vi "Realback.vi"() -> ()   [LabVIEW 2013]
uses:
  <vilib>/Utility/file.llb/Read From Spreadsheet File (DBL).vi
panel:
  in  "# skip":i32
  in  "# of sweeps":i32=1000
  out "Spectrum #":i32=999
  out "Chars":i32=1282716
  out "Fcen":dbl=213.0 format="%#_13g"
  out "# Data points":i32=101
  in  "Offset V":dbl format="%#_3g"
  out "NMR Graph + Fit":cluster{dbl, dbl}[](graph)=[{212.6, -0.16073883883883802}, {212.608, -0.16040180180180247}, {212.61599999999999, -0.1600734734734744}, {212.624, -0.1597480480480463}, {212.632, -0.1594280280280284}, {212.64, -0.15912582582582555}, {212.648, -0.15882072072072065}, {212.656, -0.158519319319321}, {212.664, -0.15823073073073043}, {212.672, -0.1579462462462453}, {212.68, -0.15766146146146215}, {212.688, -0.1573662662662664}, {212.696, -0.1570670670670683}, {212.704, -0.15675385385385404}, {212.712, -0.1564493493493483}, {212.72, -0.1561526526526524}, {212.728, -0.15587627627627706}, {212.736, -0.1556206206206206}, {212.744, -0.1553856856856856}, {212.752, -0.15515845845845858}, {212.76, -0.1549458458458459}, {212.768, -0.15473903903903835}, {212.776, -0.15453673673673607}, {212.784, -0.15433903903903998}, {212.792, -0.15414684684684804}, {212.79999999999998, -0.15395325325325318}, {212.808, -0.15376576576576428}, {212.816, -0.15358708708708604}, {212.82399999999998, -0.1534129129129131}, {212.832, -0.1532410410410411}, {212.84, -0.1530826826826821}, {212.84799999999998, -0.1529271271271264}, {212.856, -0.15278578578578608}, {212.864, -0.1526609609609621}, {212.87199999999999, -0.15253163163163322}, {212.88, -0.15241391391391546}, {212.888, -0.15231491491491583}, {212.896, -0.15221491491491465}, {212.904, -0.15212162162162043}, {212.912, -0.1520264264264249}, {212.92, -0.15195275275275122}, {212.928, -0.15188108108107995}, {212.936, -0.15181641641641605}, {212.944, -0.15176516516516494}, {212.952, -0.15173403403403407}, {212.96, -0.15173313313313336}, {212.968, -0.15177017017016978}, {212.976, -0.1518006006006003}, {212.984, -0.15173983983984016}, {212.992, -0.15169779779779818}, {213.0, -0.1516902902902905}, {213.008, -0.15169489489489518}, {213.016, -0.15168108108108158}, {213.024, -0.15169089089089133}, {213.032, -0.15172112112112154}, {213.04, -0.15176556556556584}, {213.048, -0.15179779779779762}, {213.056, -0.15185625625625562}, {213.064, -0.15193223223223107}, {213.072, -0.15198738738738587}, {213.08, -0.15204724724724555}, {213.088, -0.15212502502502398}, {213.096, -0.1522167167167166}, {213.104, -0.15231871871871952}, {213.112, -0.15243293293293445}, {213.12, -0.15255175175175337}, {213.12800000000001, -0.1526766766766775}, {213.136, -0.15282012012011958}, {213.144, -0.1529715715715709}, {213.15200000000002, -0.1531350350350349}, {213.16, -0.1533186186186189}, {213.168, -0.15351111111111057}, {213.17600000000002, -0.15370180180180038}, {213.184, -0.15391111111111092}, {213.192, -0.15412052052052155}, {213.2, -0.15434864864864928}, {213.208, -0.1545821821821811}, {213.216, -0.15481641641641614}, {213.224, -0.15505325325325345}, {213.232, -0.15529939939939943}, {213.24, -0.1555706706706705}, {213.248, -0.1558586586586596}, {213.256, -0.15617497497497437}, {213.264, -0.15652822822822776}, {213.272, -0.1569007007007014}, {213.28, -0.15727547547547563}, {213.288, -0.15764314314314382}, {213.296, -0.15800110110109958}, {213.304, -0.15834644644644752}, {213.312, -0.1587058058058067}, {213.32, -0.15907317317317304}, {213.328, -0.15945115115115094}, {213.336, -0.15984504504504424}, {213.344, -0.16024984984985124}, {213.352, -0.1606673673673666}, {213.36, -0.16110060060060055}, {213.368, -0.1615386386386386}, {213.376, -0.16198208208208292}, {213.38400000000001, -0.16242522522522437}, {213.392, -0.16287507507507482}, {213.4, -0.16338568568568626}]
  out "File size (bytes)":i32=1284000
  out "File name":string="C:\\Users\\plm\\Desktop\\rssmt\\NMR3494011168.xls"
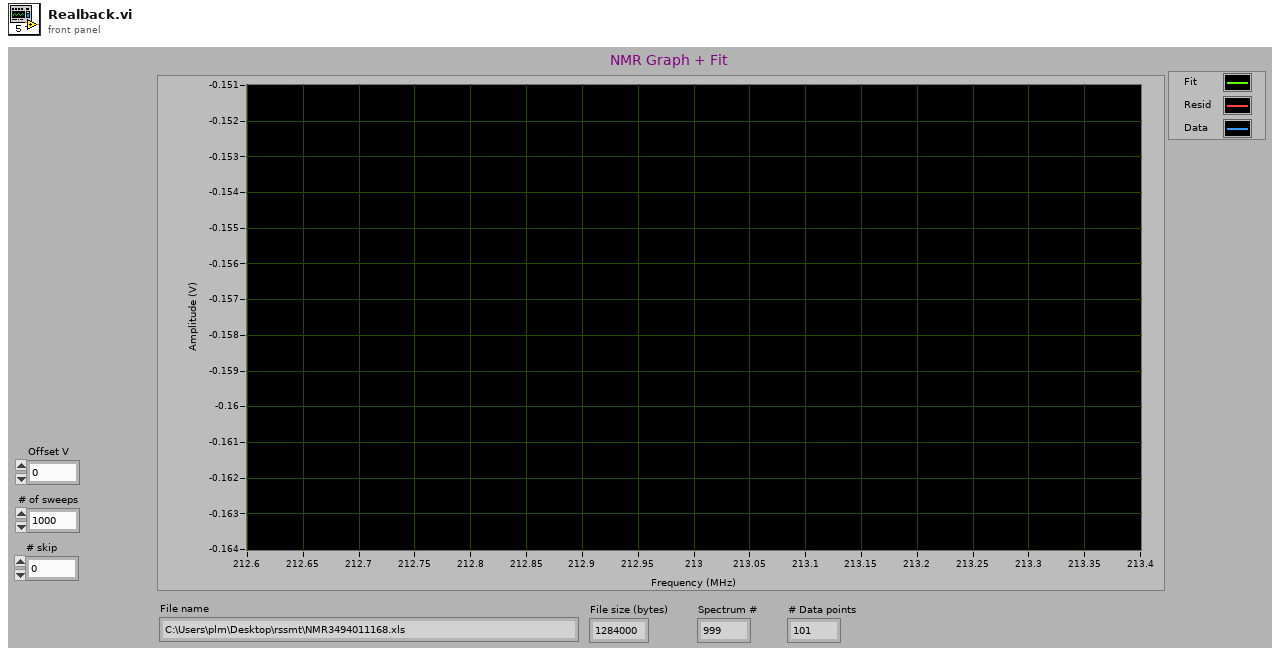
[diagram p1: front panel]
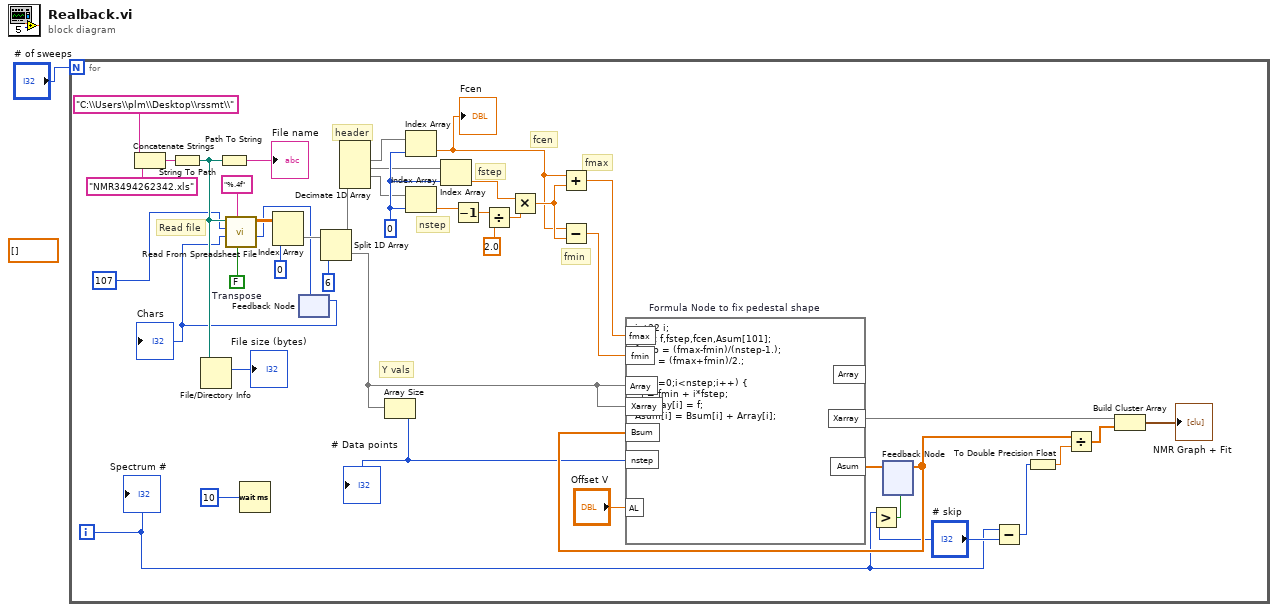
[diagram p0: block diagram]
diagram:
  (unwired) dbl[] []
  n1 = for {
    N: "# of sweeps" -> [_]
    i -> [w7]
    w26 = 0
    w40 = FALSE  # Transpose
    # "Read file"
    # "header"
    # "nstep"
    # "fstep"
    # "fcen"
    # "fmin"
    # "fmax"
    # "Y vals"
    n2 = Concatenate Strings "Concatenate Strings"("C:\\Users\\plm\\Desktop\\rssmt\\", "NMR3494262342.xls") -> (w43:string)
    n3 = String To Path(string=w43) -> (path=w39:path)
    n4 = File/Directory Info(path=w39) -> (size=→"File size (bytes)":i64)  [unwired: 1 in, 6 out]
    n5 = Path To String(path=w39) -> (string=→"File name":string)
    n6 = Wait (ms)(milliseconds to wait=10) -> ()  [unwired: 1 out]
    n7 = feedback #1() -> (w17:i32)  [unwired: 1 in]
    "Chars" <- w17
    n8 = call-poly <vilib>:"Read From Spreadsheet File.vi"("transpose (no:F)"=w40, "format (%.3f)"="%.4f", "start of read offset (chars.:0)"=w17, "number of rows (all:-1)"=107, "file path (dialog if empty)"=w39) -> ("mark after read (chars.)"=w18:i32, "all rows"=w34:dbl[][])  [unwired: 2 in, 3 out]
    n9 = Index Array "Index Array"(array=w34, index (col)=0) -> (element=w32:dbl[])  [unwired: 1 in]
    n10 = feedback-in #1(w18) -> ()
    n11 = Split 1D Array(array=w32, index=6) -> (first subarray=w35:dbl[], second subarray=w4:dbl[])
    n12 = Decimate 1D Array(w35) -> (w27:dbl[], w25:dbl[], w24:dbl[])  [unwired: 3 out]
    n13 = Array Size(array=w4) -> (size(s)=w10:i32)
    "# Data points" <- w10
    n14 = Index Array "Index Array"(array=w27, index=w26) -> (element=w19:dbl)
    "Fcen" <- w19
    n15 = Index Array(array=w24, index=w26) -> (element=w22:dbl)
    n16 = Index Array(array=w25, index=w26) -> (element=w23:dbl)
    n17 = Decrement(x=w22) -> (x-1=w31:dbl)
    n18 = Divide(x=w31, y=2.0) -> (x/y=w29:dbl)
    n19 = Multiply(x=w23, y=w29) -> (x*y=w28:dbl)
    n20 = Add(x=w19, y=w28) -> (x+y=w3:dbl)
    n21 = Subtract(x=w19, y=w28) -> (x-y=w2:dbl)
    n22 = Greater?(x=w7, y="# skip") -> (0:w9:bool)
    n23 = feedback #2() -> (w12:dbl[])  [unwired: 1 in]
    n24 = formula code="int32 i;\nfloat f,fstep,fcen,Asum[101];\nfstep = (fmax-fmin)/(nstep-1.);\nfcen = (fmax+fmin)/2.;\n\nfor (i=0;i<nstep;i++) {\n  f = fmin + i*fstep;\n  Xarray[i] = f;\nAsum[i] = Bsum[i] + Array[i];\n}" "Formula Node to fix pedestal shape"("nstep"=w10, "fmin"=w2, "fmax"=w3, "AL"="Offset V", "Array"=w4, "Xarray"=w4, "Bsum"=w12) -> ("Xarray"=w15:dbl[], "Asum"=w16:dbl[])  [unwired: 1 out]
    n25 = feedback-in #2(w16, w9) -> ()
    n26 = Subtract(x=w7, y="# skip") -> (x-y=w6:i32)
    n27 = To Double Precision Float(number=w6) -> (double precision float=w11:dbl)
    n28 = Divide(x=w12, y=w11) -> (x/y=w14:dbl[])
    n29 = Build Cluster Array ("Index & Bundle Cluster Array")(w15, w14) -> (→"NMR Graph + Fit":cluster{dbl, dbl}[])
    "Spectrum #" <- w7
  }
